vi "MW Chop PG FG.vi"() -> ()   [LabVIEW 2012]
uses:
  Microwave.lvclass
  Function Generator/Function Generator.lvclass
  Pulse Gen/Pulse Generator.lvclass
  Function Generator/Tektronix AFG 3000 Series/controls.llb/Channel.ctl
  Function Generator/Tektronix AFG 3000 Series/controls.llb/Frequency Mode.ctl
  Function Generator/Tektronix AFG 3000 Series/controls.llb/Waveform Shape.ctl
  Function Generator/Tektronix AFG 3000 Series/controls.llb/Volt Unit.ctl
  Function Generator/Tektronix AFG 3000 Series/controls.llb/Voltage.ctl
  Agilent PSG MXG Series/Agilent PSG MXG Series.lvlib
  Function Generator/Tektronix AFG 3000 Series/Tektronix AFG 3000 Series.lvlib
panel:
  in  "Enable/disable settings":bool
  in  "Copy actual to set":bool
  in  "Populate fields with member data":bool
  out "error out":errorcluster
  in  "error in (no error)":errorcluster
  in  "PG Ch 2 Sync":bool
  in  "PG Ch 1 Sync":bool
  in  "PG ch2Not rf on":bool caption="PG CH2 Not"
  in  "PG ch1Not rf on":bool caption="PG CH1 Not"
  in  "PG ch2 rf on":bool caption="PG CH2"
  in  "PG ch1 rf on":bool caption="PG CH1"
  in  "FG ch2 rf on":bool caption="FG CH2"
  in  "FG--PG":bool
  in  "FG chop freq set":dbl[unit] caption="Chop Freq."
  in  "FG volt on set":dbl[unit]=2.5 caption="On Voltage"
  in  "FG volt off set":dbl[unit] caption="Off Voltage"
  out "FG chop freq":dbl[unit] caption="Chop Freq."
  out "FG volt on":dbl[unit] caption="On Voltage"
  out "FG volt off":dbl[unit] caption="Off Voltage"
  in  "setFG":bool
  in  "FG channel":enum16{"1", "2"}(ring) caption="Channel"
  in  "FG ch1 rf on":bool caption="FG CH1"
  in  "PG chop freq set":dbl[unit]=10000.0 caption="Chop Freq."
  in  "PG volt on set":dbl[unit]=2.5 caption="On Voltage" min=-2.05 max=4.0 step=0.01
  in  "PG volt off set":dbl[unit] caption="Off Voltage" min=-2.1 max=3.95 step=0.01
  out "PG chop freq":dbl[unit] caption="Chop Freq."
  out "PG volt on":dbl[unit] caption="On Voltage"
  out "PG volt off":dbl[unit] caption="Off Voltage"
  in  "setPG":bool
  in  "PG channel":enum16{"n/a", "1", "2"}(ring)=enum."1" caption="Channel"
  in  "PG length/duty set":dbl=50.0 caption="PG pulse length/duty cycle"
  in  "PG length/duty unit set":enum16{"ns", "us", "ms", "% (duty)"}(ring)=enum."% (duty)"
  out "PG length/duty":dbl
  out "PG length/duty unit":enum16{"ns", "us", "ms", "% (duty)"}(ring)=enum."% (duty)"
  in  "readcontrol":bool
  in  "setMW":bool
  out "FG on?":bool caption="FG"
  in  "MW rf on":bool caption="MWave On/Off"
  out "MW amp":dbl=25.0 caption="MW Amp (dBm)"
  in  "MW amp set":dbl=-135.0 caption="MW Amp (dBm)"
  out "MW freq":dbl[unit] caption="MW Freq"
  in  "MW freq set":dbl[unit]=8500000000.0 caption="MW Freq"
  out "MW on?":bool caption="MW"
  out "active":bool
  in  "connect":bool
  out "PG on?":bool caption="PG"
  in  "exit":bool
  in  "read":bool
  # "Microwave Modulation"
  # "Set Chop via Pulse Generator or Function Generator and PIN Diode"
  # "Pulse Generator"
  # "Function Generator"
  # "(ready when\nblinking)"
  # "Outputs"
  # "Outputs"
  # "Microwaves"
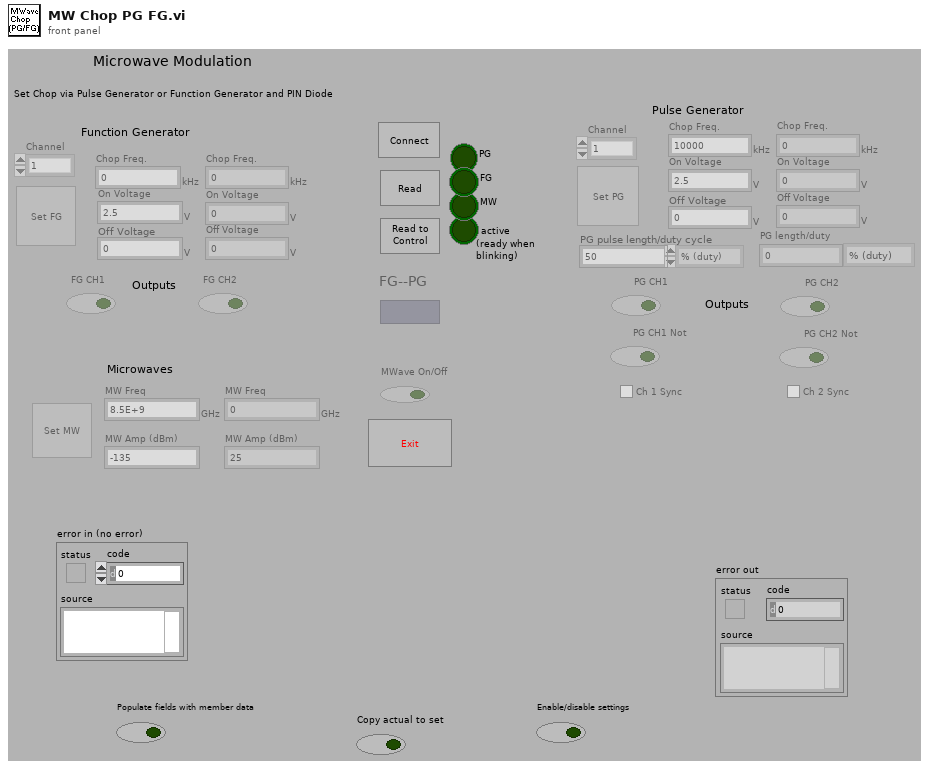
[diagram p1: front panel]
types:
  T1 = enum16{"CW", "Fixed", "Stepped Sweep", "List Sweep"}
  T2 = typedef "Voltage.ctl" = enum16{"amplitude", "offset", "high", "low", "high limit", "low limit"}
  T3 = typedef "Volt Unit.ctl" = enum16{"VPP", "VRMS", "DBM"}
  T4 = typedef "Frequency Mode.ctl" = enum16{"CW", "Sweep"}
  T5 = typedef "Channel.ctl" = u16
  T6 = typedef "Waveform Shape.ctl" = u16
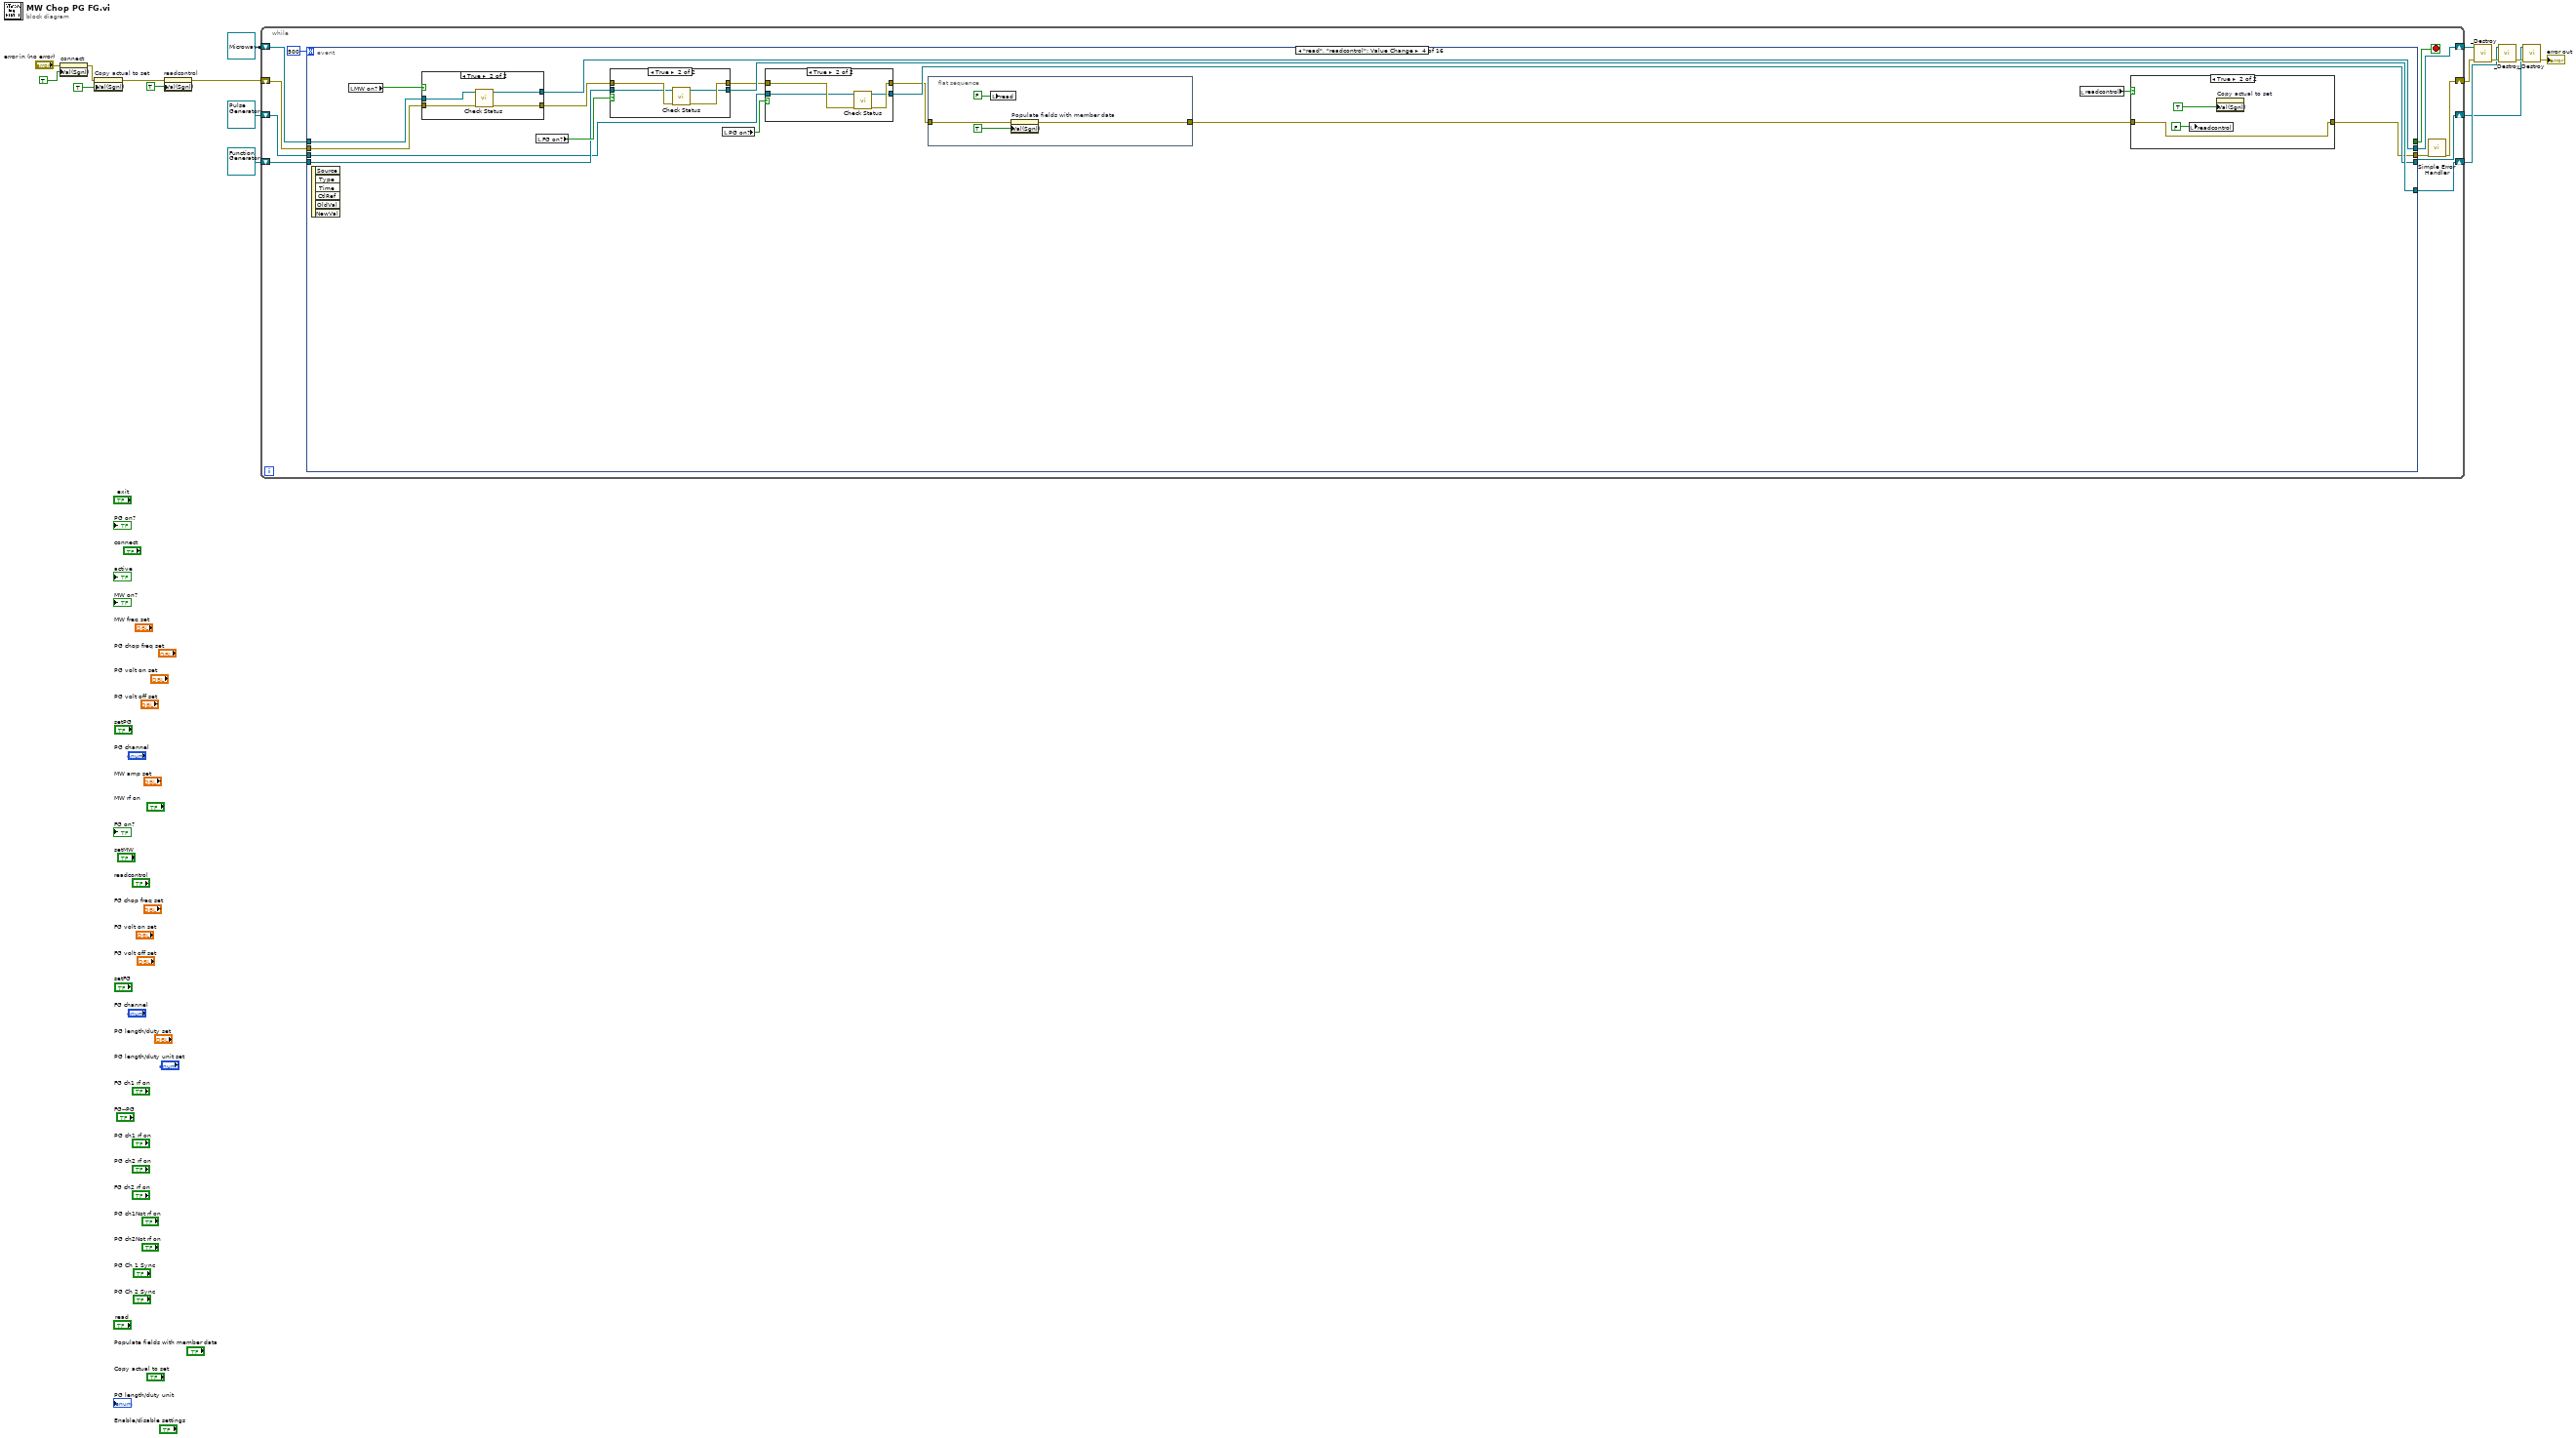
[diagram p0: block diagram]
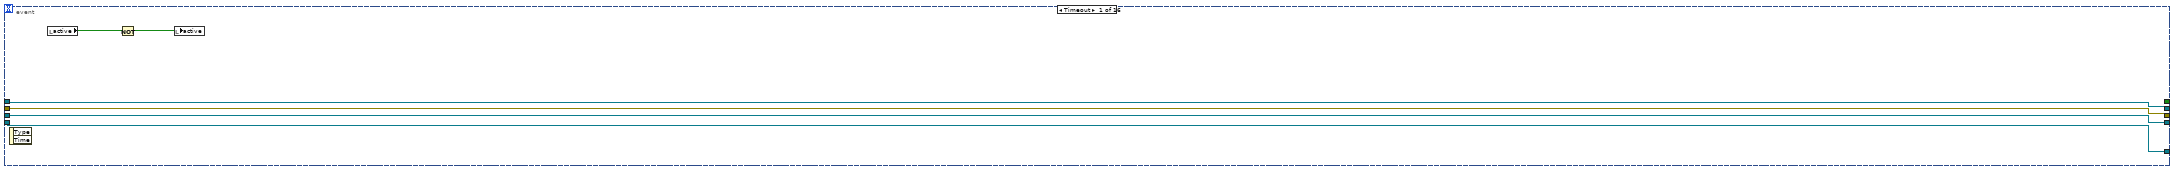
[diagram p2: hidden frame]
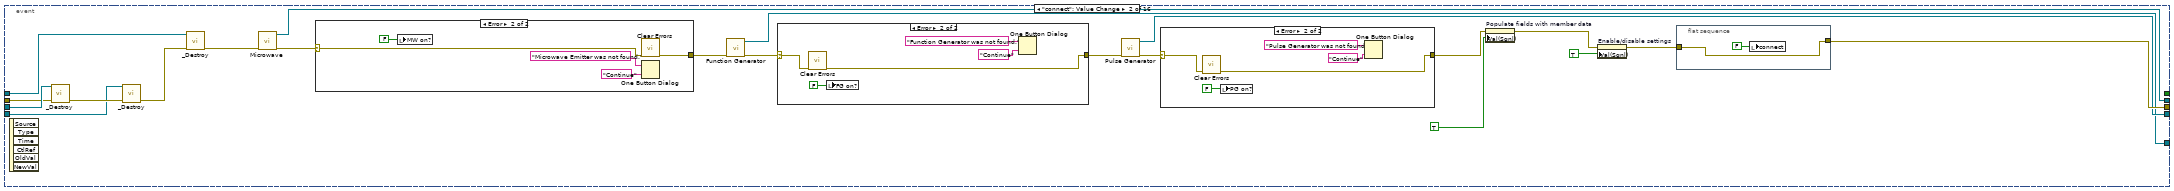
[diagram p3: hidden frame]
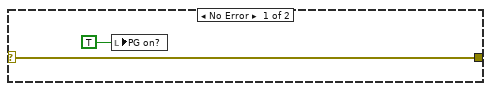
[diagram p4: hidden frame]
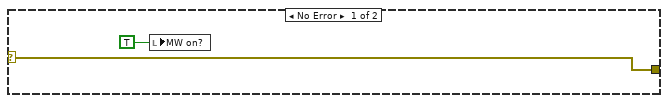
[diagram p5: hidden frame]
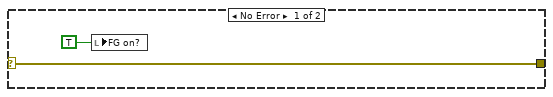
[diagram p6: hidden frame]
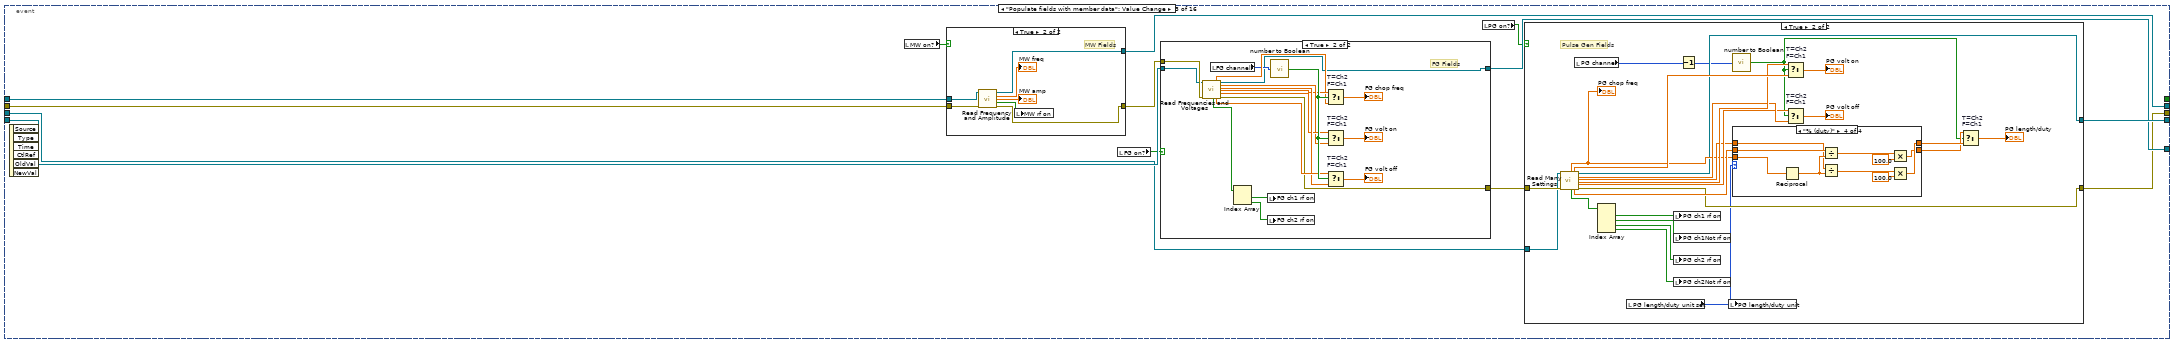
[diagram p7: hidden frame]
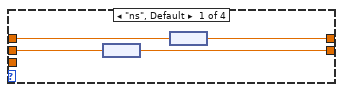
[diagram p9: hidden frame]
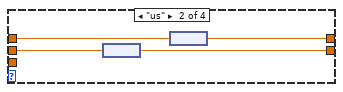
[diagram p10: hidden frame]
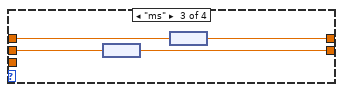
[diagram p11: hidden frame]
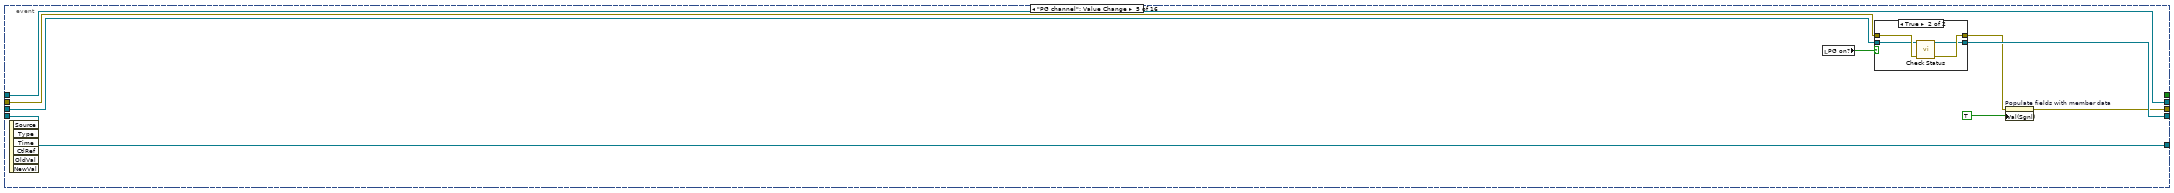
[diagram p18: hidden frame]
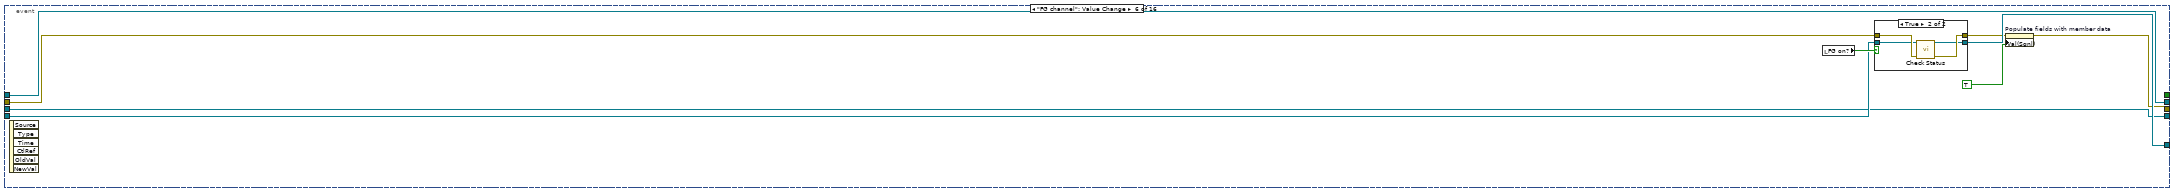
[diagram p20: hidden frame]
diagram:
  n1 = property on="connect" class="Bool (strict)"(error in="error in (no error)", "Val(Sgnl)"=TRUE ("Value (Signaling)")) -> (error out=w12:errorcluster)  [unwired: 1 in, 1 out]
  n2 = property on="Copy actual to set" class="Bool (strict)"(error in=w12, "Val(Sgnl)"=TRUE ("Value (Signaling)")) -> (error out=w3:errorcluster)  [unwired: 1 in, 1 out]
  n3 = property on="readcontrol" class="Bool (strict)"(error in=w3, "Val(Sgnl)"=TRUE ("Value (Signaling)")) -> (error out=w2:errorcluster)  [unwired: 1 in, 1 out]
  n4 = while {
    shift-right: [w21] -> w4
    shift-left: w2 -> [w22]
    shift-right: [w19] -> w7
    shift-left: refnum<class "Microwave.lvclass"> refnum ("Microwave out") -> [w25]
    shift-right: [w18] -> w6
    shift-left: refnum<class "Function Generator.lvclass"> refnum ("Function Generator out") -> [w24]
    shift-right: [w20] -> w5
    shift-left: refnum<class "Pulse Generator.lvclass"> refnum ("Pulse Generator out") -> [w23]
    stop <- w26 stop-if-true
    n5 = event shown="[3] \"read\", \"readcontrol\": Value Change" {
      selector: _ -> [_ _ _ _ _ _ _ _ _ _ _ _ _ _ _ _]
      dyn-events: _ -> [_ _ _ _ _ _ _ _ _ _ _ _ _ _ _ _]
      timeout: 500 -> [_ _ _ _ _ _ _ _ _ _ _ _ _ _ _ _]
      tunnel: w22 -> [w29 w43 w89 w181 w214 w232 w245 w267 w291 w310 w332 w360 w458 w497 w501 w520]
      tunnel: [w29 w41 w84 w170 w216 w227 w245 w258 w273 w309 w331 w365 w453 w497 w498 w520] -> w27
      tunnel: [_ _ _ _ _ _ _ _ _ _ _ _ _ TRUE ("exit") _ _] -> w26
      tunnel: w25 -> [w32 w45 w90 w182 w215 w231 w244 w262 w300 w328 w330 w362 w457 w496 w507 w519]
      tunnel: w24 -> [w31 w46 w88 w178 w213 w234 w243 w272 w297 w327 w334 w364 w455 w495 w506 w518]
      tunnel: w23 -> [w30 w47 w87 w175 w219 w229 w242 w271 w299 w312 w333 w361 w456 w494 w505 w517]
      tunnel: [w32 w39 w91 w180 w215 w231 w244 w257 w300 w328 w329 w362 w457 w496 w507 w519] -> w19
      tunnel: [w31 w38 w85 w177 w213 w233 w243 w272 w275 w327 w334 w364 w454 w495 w506 w518] -> w18
      tunnel: [w30 w40 w86 w174 w218 w229 w242 w271 w299 w311 w333 w359 w456 w494 w505 w517] -> w20
      event Timeout {
        n6 = event-data() -> ()  [unwired: 3 out]
        n7 = local read "active"() -> (w33:bool)
        n8 = Not(x=w33) -> (.not. x?=w34:bool)
        n9 = local write "active"(w34) -> ()
      }
      event "connect": Value Change {
        n10 = event-data() -> ()  [unwired: 7 out]
        n11 = call-dynamic "_Destroy.vi"("error in (no error)"=w43, "Instrument in"=w47) -> ("error out"=w50:errorcluster)  [unwired: 9 out]
        n12 = call-dynamic "_Destroy.vi"("error in (no error)"=w50, "Instrument in"=w46) -> ("error out"=w49:errorcluster)  [unwired: 9 out]
        n13 = call-dynamic "_Destroy.vi"("error in (no error)"=w49, "Instrument in"=w45) -> ("error out"=w48:errorcluster)  [unwired: 9 out]
        n14 = call "Microwave.vi"("error in (no error)"=w48) -> ("error out"=w51:errorcluster, "Microwave out"=w39:refnum<class "Microwave.lvclass">)  [unwired: 9 out]
        n15 = case shown="Error" w51 {
          selector: w51 -> [w65 w70]
          tunnel: [w65 w69] -> w54
          frame No Error {
            n16 = local write "MW on?"(TRUE ("FGon")) -> ()
          }
          frame Error {
            n17 = local write "MW on?"(FALSE ("FGon")) -> ()
            n18 = call <vilib>:"Clear Errors.vi"("error in (no error)"=w70) -> ("error out"=w69:errorcluster)  [unwired: 6 out]
            n19 = One Button Dialog(message="Microwave Emitter was not found.", button name ("OK")="Continue") -> ()  [unwired: 1 out]
          }
        }
        n20 = call "Function Generator.vi"("error in (no error)"=w54) -> ("error out"=w52:errorcluster, "Function Generator out"=w38:refnum<class "Function Generator.lvclass">)  [unwired: 9 out]
        n21 = case shown="Error" w52 {
          selector: w52 -> [w72 w77]
          tunnel: [w72 w76] -> w55
          frame No Error {
            n22 = local write "FG on?"(TRUE ("FGon")) -> ()
          }
          frame Error {
            n23 = call <vilib>:"Clear Errors.vi"("error in (no error)"=w77) -> ("error out"=w76:errorcluster)  [unwired: 6 out]
            n24 = local write "FG on?"(FALSE ("FGon")) -> ()
            n25 = One Button Dialog(message="Function Generator was not found.", button name ("OK")="Continue") -> ()  [unwired: 1 out]
          }
        }
        n26 = call "Pulse Generator.vi"("error in (no error)"=w55) -> ("error out"=w53:errorcluster, "Pulse Generator out"=w40:refnum<class "Pulse Generator.lvclass">)  [unwired: 9 out]
        n27 = case shown="Error" w53 {
          selector: w53 -> [w58 w63]
          tunnel: [w58 w62] -> w36
          frame No Error {
            n28 = local write "PG on?"(TRUE ("FGon")) -> ()
          }
          frame Error {
            n29 = call <vilib>:"Clear Errors.vi"("error in (no error)"=w63) -> ("error out"=w62:errorcluster)  [unwired: 6 out]
            n30 = local write "PG on?"(FALSE ("FGon")) -> ()
            n31 = One Button Dialog(message="Pulse Generator was not found.", button name ("OK")="Continue") -> ()  [unwired: 1 out]
          }
        }
        n32 = property on="Populate fields with member data" class="Bool (strict)"(error in=w36, "Val(Sgnl)"=TRUE ("Value (Signaling)")) -> (error out=w37:errorcluster)  [unwired: 1 in, 1 out]
        n33 = property on="Enable/disable settings" class="Bool (strict)"(error in=w37, "Val(Sgnl)"=TRUE ("Value (Signaling)")) -> (error out=w42:errorcluster)  [unwired: 1 in, 1 out]
        n34 = flat-sequence {
          tunnel: [w56] -> w41
          tunnel: w42 -> [w56]
          frame #0 {
            n35 = local write "connect"(FALSE) -> ()
          }
        }
      }
      event "Populate fields with member data": Value Change {
        n36 = event-data() -> ()  [unwired: 7 out]
        n37 = local read "MW on?"() -> (w81:bool)
        n38 = case shown="True" w81 {
          tunnel: w90 -> [w162 w163]
          tunnel: w89 -> [w161 w167]
          tunnel: [w161 w164] -> w83
          tunnel: [w162 w166] -> w91
          frame False {
          }
          frame True {
            # "MW Fields"
            n39 = call-dynamic "Read Frequency and Amplitude.vi"("Microwave.lvclass in"=w163, "error in (no error)"=w167) -> ("Microwave.lvclass out"=w166:refnum<class "Microwave.lvclass">, "Frequency"=→"MW freq":dbl[unit], "Amplitude (dBm)"=→"MW amp":dbl, "rf on?"=w165:bool, "error out"=w164:errorcluster)  [unwired: 9 out]
            n40 = local write "MW rf on"(w165) -> ()
          }
        }
        n41 = local read "FG on?"() -> (w80:bool)
        n42 = case shown="True" w80 {
          tunnel: w83 -> [w142 w149]
          tunnel: [w142 w148] -> w82
          tunnel: [w141 w147] -> w85
          tunnel: w88 -> [w141 w146]
          frame False {
          }
          frame True {
            # "FG Fields"
            n43 = call-dynamic "Read Frequencies and Voltages.vi"("Function Generator.lvclass in"=w146, "error in (no error)"=w149) -> ("array of outputs on"=w145:bool[], "Ch1 Frequency"=w151:dbl[unit], "Ch2 Low"=w158:dbl[unit], "Function Generator.lvclass out"=w147:refnum<class "Function Generator.lvclass">, "Ch1 High"=w154:dbl[unit], "Ch1 Low"=w157:dbl[unit], "Ch2 Frequency"=w152:dbl[unit], "Ch2 High"=w155:dbl[unit], "error out"=w148:errorcluster)  [unwired: 9 out]
            n44 = local read "FG channel"() -> (w150:enum16{"1", "2"})
            n45 = Index Array(array=w145) -> (element #1=w144:bool, element #2=w143:bool)  [unwired: 2 in]
            n46 = local write "FG ch1 rf on"(w144) -> ()
            n47 = local write "FG ch2 rf on"(w143) -> ()
            n48 = call "number to Boolean.vi"("Numeric"=w150) -> ("Boolean"=w159:bool)
            n49 = Select "T=Ch2\nF=Ch1"(t=w152, s=w159, f=w151) -> (s? t:f=→"FG chop freq":dbl[unit])
            n50 = Select "T=Ch2\nF=Ch1"(t=w155, s=w159, f=w154) -> (s? t:f=→"FG volt on":dbl[unit])
            n51 = Select "T=Ch2\nF=Ch1"(t=w158, s=w159, f=w157) -> (s? t:f=→"FG volt off":dbl[unit])
          }
        }
        n52 = local read "PG on?"() -> (w79:bool)
        n53 = case shown="True" w79 {
          tunnel: w82 -> [w92 w104]
          tunnel: [w92 w103] -> w84
          tunnel: w87 -> [w93 w96]
          tunnel: [w93 w102] -> w86
          frame False {
          }
          frame True {
            # "Pulse Gen Fields"
            n54 = call-dynamic "Read Many Settings.vi"("Pulse Generator.lvclass in"=w96, "error in (no error)"=w104) -> ("Overall Frequency"=w105:dbl[unit], "Outputs 1/!1/2/!2"=w97:bool[], "Output Levels.1 High"=w117:dbl[unit], "Ch2Width"=w108:dbl[unit], "Pulse Generator.lvclass out"=w102:refnum<class "Pulse Generator.lvclass">, "Output Levels.1 Low"=w114:dbl[unit], "Ch1Width"=w110:dbl[unit], "Output Levels.2 High"=w116:dbl[unit], "Output Levels.2 Low"=w113:dbl[unit], "error out"=w103:errorcluster)  [unwired: 8 out]
            "PG chop freq" <- w105
            n55 = local read "PG channel"() -> (w118:enum16{"n/a", "1", "2"})
            n56 = Index Array(array=w97) -> (element #1=w101:bool, element #2=w100:bool, element #3=w99:bool, element #4=w98:bool)  [unwired: 4 in]
            n57 = local read "PG length/duty unit set"() -> (w95:enum16{"ns", "us", "ms", "% (duty)"})
            n58 = local write "PG ch1 rf on"(w101) -> ()
            n59 = local write "PG ch1Not rf on"(w100) -> ()
            n60 = local write "PG ch2 rf on"(w99) -> ()
            n61 = local write "PG ch2Not rf on"(w98) -> ()
            n62 = Decrement(x=w118) -> (x-1=w94:enum16{"n/a", "1", "2"})
            n63 = local write "PG length/duty unit"(w95) -> ()
            n64 = call "number to Boolean.vi"("Numeric"=w94) -> ("Boolean"=w106:bool)
            n65 = case shown="\"% (duty)\"" w95 {
              tunnel: [w121 w124 w127 w132] -> w111
              tunnel: w110 -> [w122 w125 w128 w135]
              tunnel: w108 -> [w120 w126 w130 w137]
              tunnel: [w119 w123 w129 w131] -> w107
              tunnel: w105 -> [_ _ _ w140]
              frame "ns", Default {
                n66 = node(w120) -> (w119:dbl)
                n67 = node(w122) -> (w121:dbl)
              }
              frame "us" {
                n68 = node(w126) -> (w123:dbl)
                n69 = node(w125) -> (w124:dbl)
              }
              frame "ms" {
                n70 = node(w130) -> (w129:dbl)
                n71 = node(w128) -> (w127:dbl)
              }
              frame "% (duty)" {
                n72 = Reciprocal(x=w140) -> (1/x=w136:dbl[unit])
                n73 = Divide(x=w137, y=w136) -> (x/y=w138:dbl)
                n74 = Divide(x=w135, y=w136) -> (x/y=w133:dbl)
                n75 = Multiply(x=w138, y=100.0) -> (x*y=w131:dbl)
                n76 = Multiply(x=w133, y=100.0) -> (x*y=w132:dbl)
              }
            }
            n77 = Select "T=Ch2\nF=Ch1"(t=w116, s=w106, f=w117) -> (s? t:f=→"PG volt on":dbl[unit])
            n78 = Select "T=Ch2\nF=Ch1"(t=w113, s=w106, f=w114) -> (s? t:f=→"PG volt off":dbl[unit])
            n79 = Select "T=Ch2\nF=Ch1"(t=w107, s=w106, f=w111) -> (s? t:f=→"PG length/duty":dbl)
          }
        }
      }
      event "read", "readcontrol": Value Change {
        n80 = event-data() -> ()  [unwired: 7 out]
        n81 = local read "MW on?"() -> (w185:bool)
        n82 = case shown="True" w185 {
          tunnel: w182 -> [w206 w211]
          tunnel: w181 -> [w207 w210]
          tunnel: [w206 w209] -> w180
          tunnel: [w207 w208] -> w179
          frame False {
          }
          frame True {
            n83 = call-dynamic "Check Status.vi"("error in (no error)"=w210, "Microwave in"=w211) -> ("error out"=w208:errorcluster, "Microwave out"=w209:refnum<class "Microwave.lvclass">)  [unwired: 8 out]
          }
        }
        n84 = local read "FG on?"() -> (w184:bool)
        n85 = case shown="True" w184 {
          tunnel: w179 -> [w200 w205]
          tunnel: [w200 w204] -> w176
          tunnel: w178 -> [w201 w203]
          tunnel: [w201 w202] -> w177
          frame False {
          }
          frame True {
            n86 = call-dynamic "Check Status.vi"("error in (no error)"=w205, "Function Generator in"=w203) -> ("error out"=w204:errorcluster, "Function Generator out"=w202:refnum<class "Function Generator.lvclass">)  [unwired: 8 out]
          }
        }
        n87 = local read "PG on?"() -> (w183:bool)
        n88 = case shown="True" w183 {
          tunnel: w176 -> [w194 w199]
          tunnel: [w194 w198] -> w173
          tunnel: w175 -> [w195 w197]
          tunnel: [w195 w196] -> w174
          frame False {
          }
          frame True {
            n89 = call-dynamic "Check Status.vi"("error in (no error)"=w199, "Pulse Generator in"=w197) -> ("error out"=w198:errorcluster, "Pulse Generator out"=w196:refnum<class "Pulse Generator.lvclass">)  [unwired: 8 out]
          }
        }
        n90 = flat-sequence {
          tunnel: w173 -> [w193]
          tunnel: [w190] -> w171
          frame #0 {
            n91 = local write "read"(FALSE ("read")) -> ()
            n92 = property on="Populate fields with member data" class="Bool (strict)"(error in=w193, "Val(Sgnl)"=TRUE ("Value (Signaling)")) -> (error out=w190:errorcluster)  [unwired: 1 in, 1 out]
          }
        }
        n93 = local read "readcontrol"() -> (w172:bool)
        n94 = case shown="True" w172 {
          tunnel: [w186 w187] -> w170
          tunnel: w171 -> [w186 w187]
          frame False {
          }
          frame True {
            n95 = local write "readcontrol"(FALSE ("readcontrol")) -> ()
            n96 = property on="Copy actual to set" class="Bool (strict)"("Val(Sgnl)"=TRUE ("Value (Signaling)")) -> ()  [unwired: 2 in, 2 out]
          }
        }
      }
      event "PG channel": Value Change {
        n97 = event-data() -> ()  [unwired: 7 out]
        n98 = local read "PG on?"() -> (w220:bool)
        n99 = case shown="True" w220 {
          tunnel: w214 -> [w221 w226]
          tunnel: [w221 w225] -> w217
          tunnel: w219 -> [w222 w224]
          tunnel: [w222 w223] -> w218
          frame False {
          }
          frame True {
            n100 = call-dynamic "Check Status.vi"("error in (no error)"=w226, "Pulse Generator in"=w224) -> ("error out"=w225:errorcluster, "Pulse Generator out"=w223:refnum<class "Pulse Generator.lvclass">)  [unwired: 8 out]
          }
        }
        n101 = property on="Populate fields with member data" class="Bool (strict)"(error in=w217, "Val(Sgnl)"=TRUE ("Value (Signaling)")) -> (error out=w216:errorcluster)  [unwired: 1 in, 1 out]
      }
      event "FG channel": Value Change {
        n102 = event-data() -> ()  [unwired: 7 out]
        n103 = local read "FG on?"() -> (w235:bool)
        n104 = case shown="True" w235 {
          tunnel: w232 -> [w236 w241]
          tunnel: [w236 w240] -> w230
          tunnel: w234 -> [w237 w239]
          tunnel: [w237 w238] -> w233
          frame False {
          }
          frame True {
            n105 = call-dynamic "Check Status.vi"("error in (no error)"=w241, "Function Generator in"=w239) -> ("error out"=w240:errorcluster, "Function Generator out"=w238:refnum<class "Function Generator.lvclass">)  [unwired: 8 out]
          }
        }
        n106 = property on="Populate fields with member data" class="Bool (strict)"(error in=w230, "Val(Sgnl)"=TRUE ("Value (Signaling)")) -> (error out=w227:errorcluster)  [unwired: 1 in, 1 out]
      }
      event "Copy actual to set": Value Change {
        n107 = event-data() -> ()  [unwired: 7 out]
        n108 = flat-sequence {
          frame #0 {
            n109 = local read "MW freq"() -> (w246:dbl[unit])
            n110 = local read "MW amp"() -> (w247:dbl)
            n111 = local write "MW freq set"(w246) -> ()
            n112 = local write "MW amp set"(w247) -> ()
          }
          frame #1 {
            n113 = local read "FG chop freq"() -> (w250:dbl[unit])
            n114 = local read "FG volt off"() -> (w248:dbl[unit])
            n115 = local read "FG volt on"() -> (w249:dbl[unit])
            n116 = local write "FG chop freq set"(w250) -> ()
            n117 = local write "FG volt on set"(w249) -> ()
            n118 = local write "FG volt off set"(w248) -> ()
          }
          frame #2 {
            n119 = local read "PG length/duty"() -> (w254:dbl)
            n120 = local read "PG chop freq"() -> (w251:dbl[unit])
            n121 = local read "PG volt off"() -> (w252:dbl[unit])
            n122 = local read "PG volt on"() -> (w253:dbl[unit])
            n123 = local read "PG length/duty unit"() -> (w255:enum16{"ns", "us", "ms", "% (duty)"})
            n124 = local write "PG volt off set"(w252) -> ()
            n125 = local write "PG length/duty set"(w254) -> ()
            n126 = local write "PG chop freq set"(w251) -> ()
            n127 = local write "PG volt on set"(w253) -> ()
            n128 = local write "PG length/duty unit set"(w255) -> ()
          }
        }
      }
      event "MW rf on": Value Change {
        n129 = event-data() -> ("NewVal"=w261:bool)  [unwired: 6 out]
        n130 = call-dynamic "VISA Get Session.vi"("error in (no error)"=w267, "Instrument.lvclass in"=w262) -> ("error out"=w270:errorcluster, "VISA Resource Name"=w266:refnum<visa-resource-name>, "Instrument.lvclass out"=w263:refnum<class "Microwave.lvclass">)  [unwired: 7 out]
        n131 = call "Set Output.vi"("error in (no error)"=w270, "Output On"=w261, "VISA resource name"=w266) -> ("error out"=w269:errorcluster, "VISA resource name out"=w265:refnum<visa-resource-name>)  [unwired: 7 out]
        n132 = call "Query Output.vi"("error in (no error)"=w269, "VISA resource name"=w265) -> ("error out"=w268:errorcluster, "Output On?"=w260:bool, "VISA resource name out"=w264:refnum<visa-resource-name>)  [unwired: 7 out]
        n133 = local write "MW rf on"(w260) -> ()
        n134 = call-dynamic "VISA Save Session.vi"("error in (no error)"=w268, "VISA Resource Name"=w264, "Instrument.lvclass in"=w263) -> ("error out"=w259:errorcluster, "Instrument.lvclass out"=w256:refnum<class "Microwave.lvclass">)  [unwired: 7 out]
        n135 = call-dynamic "Set member data - output.vi"("error in (no error)"=w259, "rf on?"=w260, "Microwave.lvclass in"=w256) -> ("error out"=w258:errorcluster, "Microwave.lvclass out"=w257:refnum<class "Microwave.lvclass">)  [unwired: 7 out]
      }
      event "FG ch1 rf on", "FG ch2 rf on": Value Change {
        w282 = T5 1 items=["Channel 1", "Channel 2"] ("Channel (0: Channel 1)")
        w283 = T5 1 items=["Channel 1", "Channel 2"] ("Channel (0: Channel 1)")
        w284 = T5 0 items=["Channel 1", "Channel 2"] ("Channel (0: Channel 1)")
        w285 = T5 0 items=["Channel 1", "Channel 2"] ("Channel (0: Channel 1)")
        n136 = event-data() -> ()  [unwired: 7 out]
        n137 = local read "FG ch1 rf on"() -> (w281:bool)
        n138 = call-dynamic "VISA Get Session.vi"("error in (no error)"=w291, "Instrument.lvclass in"=w297) -> ("error out"=w296:errorcluster, "VISA Resource Name"=w290:refnum<visa-resource-name>, "Instrument.lvclass out"=w298:refnum<class "Function Generator.lvclass">)  [unwired: 7 out]
        n139 = call "Enable Output.vi"("Enable Output (T: Enable)"=w281, "error in (no error)"=w296, "Channel (0: Channel 1)"=w285, "VISA resource name"=w290) -> ("error out"=w295:errorcluster, "VISA resource name out"=w289:refnum<visa-resource-name>)  [unwired: 6 out]
        n140 = local read "FG ch2 rf on"() -> (w280:bool)
        n141 = call "Query Output.vi"("error in (no error)"=w295, "Channel (0: Channel 1)"=w284, "VISA resource name"=w289) -> ("error out"=w294:errorcluster, "Output Enabled?"=w279:bool, "VISA resource name out"=w288:refnum<visa-resource-name>)  [unwired: 6 out]
        n142 = local write "FG ch1 rf on"(w279) -> ()
        n143 = call "Enable Output.vi"("Enable Output (T: Enable)"=w280, "error in (no error)"=w294, "Channel (0: Channel 1)"=w283, "VISA resource name"=w288) -> ("error out"=w293:errorcluster, "VISA resource name out"=w287:refnum<visa-resource-name>)  [unwired: 6 out]
        n144 = call "Query Output.vi"("error in (no error)"=w293, "Channel (0: Channel 1)"=w282, "VISA resource name"=w287) -> ("error out"=w292:errorcluster, "Output Enabled?"=w278:bool, "VISA resource name out"=w286:refnum<visa-resource-name>)  [unwired: 6 out]
        n145 = local write "FG ch2 rf on"(w278) -> ()
        n146 = call-dynamic "VISA Save Session.vi"("error in (no error)"=w292, "VISA Resource Name"=w286, "Instrument.lvclass in"=w298) -> ("error out"=w274:errorcluster, "Instrument.lvclass out"=w276:refnum<class "Function Generator.lvclass">)  [unwired: 7 out]
        n147 = Build Array(w279, w278) -> (w277:bool[])
        n148 = call-dynamic "Set member data - outputs on.vi"("error in (no error)"=w274, "Array of outputs on?"=w277, "Function Generator.lvclass in"=w276) -> ("error out"=w273:errorcluster, "Function Generator.lvclass out"=w275:refnum<class "Function Generator.lvclass">)  [unwired: 7 out]
      }
      event "PG ch1 rf on", "PG ch1Not rf on", "PG ch2 rf on", "PG ch2Not rf on": Value Change {
        n149 = event-data() -> ()  [unwired: 7 out]
        n150 = local read "PG ch1Not rf on"() -> (w306:bool)
        n151 = local read "PG ch2Not rf on"() -> (w302:bool)
        n152 = local read "PG Ch 1 Sync"() -> (w308:bool)
        n153 = local read "PG Ch 2 Sync"() -> (w304:bool)
        n154 = local read "PG ch1 rf on"() -> (w305:bool)
        n155 = local read "PG ch2 rf on"() -> (w301:bool)
        n156 = Select(t=w305, s=w308, f=w306) -> (s? t:f=w307:bool)
        n157 = Select(t=w301, s=w304, f=w302) -> (s? t:f=w303:bool)
        n158 = call-dynamic "VISA Get Session.vi"("error in (no error)"=w310, "Instrument.lvclass in"=w312) -> ("error out"=w322:errorcluster, "VISA Resource Name"=w325:refnum<visa-resource-name>, "Instrument.lvclass out"=w326:refnum<class "Pulse Generator.lvclass">)  [unwired: 7 out]
        n159 = call "HP81110A Output Set - Fast.vi"("notoutput2"=w303, "output1"=w305, "error in (no error)"=w322, "output2"=w301, "notoutput1"=w307, "VISA session"=w325) -> ("error out"=w321:errorcluster, "dup VISA session"=w324:refnum<visa-resource-name>)  [unwired: 4 out]
        n160 = call "HP81110A Output Get.vi"("error in (no error)"=w321, "VISA session"=w324) -> ("error out"=w320:errorcluster, "output2OUT"=w317:bool, "notoutput1OUT"=w318:bool, "dup VISA session"=w323:refnum<visa-resource-name>, "notoutput2OUT"=w316:bool, "output1OUT"=w319:bool)  [unwired: 4 out]
        n161 = local write "PG ch1 rf on"(w319) -> ()
        n162 = local write "PG ch1Not rf on"(w318) -> ()
        n163 = local write "PG ch2 rf on"(w317) -> ()
        n164 = local write "PG ch2Not rf on"(w316) -> ()
        n165 = Build Array(w319, w318, w317, w316) -> (w315:bool[])
        n166 = call-dynamic "VISA Save Session.vi"("error in (no error)"=w320, "VISA Resource Name"=w323, "Instrument.lvclass in"=w326) -> ("error out"=w313:errorcluster, "Instrument.lvclass out"=w314:refnum<class "Pulse Generator.lvclass">)  [unwired: 7 out]
        n167 = call-dynamic "Set member data - outputs on.vi"("error in (no error)"=w313, "Outputs 1/!1/2/!2"=w315, "Pulse Generator.lvclass in"=w314) -> ("error out"=w309:errorcluster, "Pulse Generator.lvclass out"=w311:refnum<class "Pulse Generator.lvclass">)  [unwired: 7 out]
      }
      event "setMW": Value Change {
        n168 = event-data() -> ()  [unwired: 7 out]
        n169 = flat-sequence {
          tunnel: w332 -> [w344]
          tunnel: w330 -> [w343]
          tunnel: [w338] -> w331
          tunnel: [w336] -> w329
          frame #0 {
            n170 = call-dynamic "VISA Get Session.vi"("error in (no error)"=w344, "Instrument.lvclass in"=w343) -> ("error out"=w357:errorcluster, "VISA Resource Name"=w355:refnum<visa-resource-name>, "Instrument.lvclass out"=w356:refnum<class "Microwave.lvclass">)  [unwired: 7 out]
            n171 = call "Set Frequency Mode.vi"("error in (no error)"=w357, "Frequency Mode"=T1."CW", "VISA resource name"=w355) -> ("error out"=w348:errorcluster, "VISA resource name out"=w347:refnum<visa-resource-name>)  [unwired: 7 out]
            n172 = local read "MW freq set"() -> (w350:dbl[unit])
            n173 = call "Set Amplitude Mode.vi"("error in (no error)"=w348, "Amplitude Mode"=enum16{"Fixed", "Stepped Sweep", "List Sweep"}."Fixed", "VISA resource name"=w347) -> ("error out"=w351:errorcluster, "VISA resource name out"=w349:refnum<visa-resource-name>)  [unwired: 7 out]
            n174 = local read "MW amp set"() -> (w352:dbl)
            n175 = call "Set Frequency.vi"("error in (no error)"=w351, "Frequency"=w350, "VISA resource name"=w349) -> ("error out"=w353:errorcluster, "VISA resource name out"=w354:refnum<visa-resource-name>)  [unwired: 7 out]
            n176 = call "Set Amplitude.vi"("error in (no error)"=w353, "Amplitude (dBm)"=w352, "VISA resource name"=w354) -> ("error out"=w342:errorcluster, "VISA resource name out"=w341:refnum<visa-resource-name>)  [unwired: 7 out]
            n177 = call-dynamic "VISA Save Session.vi"("error in (no error)"=w342, "VISA Resource Name"=w341, "Instrument.lvclass in"=w356) -> ("error out"=w340:errorcluster, "Instrument.lvclass out"=w337:refnum<class "Microwave.lvclass">)  [unwired: 7 out]
            n178 = call-dynamic "Check Status.vi"("error in (no error)"=w340, "Microwave in"=w337) -> ("error out"=w339:errorcluster, "Microwave out"=w336:refnum<class "Microwave.lvclass">)  [unwired: 8 out]
            n179 = property on="Populate fields with member data" class="Bool (strict)"(error in=w339, "Val(Sgnl)"=TRUE ("Value (Signaling)")) -> (error out=w338:errorcluster)  [unwired: 1 in, 1 out]
          }
          frame #1 {
            n180 = local write "setMW"(FALSE) -> ()
          }
        }
      }
      event "setPG": Value Change {
        n181 = event-data() -> ()  [unwired: 7 out]
        n182 = flat-sequence {
          tunnel: [w368] -> w363
          tunnel: w361 -> [w385]
          tunnel: w360 -> [w384]
          tunnel: [w366] -> w359
          tunnel: [w451] -> w365
          tunnel: w363 -> [w451]
          frame #0 {
            n183 = local read "PG volt off set"() -> (w393:dbl[unit])
            n184 = local read "PG volt on set"() -> (w394:dbl[unit])
            n185 = call-dynamic "VISA Get Session.vi"("error in (no error)"=w384, "Instrument.lvclass in"=w385) -> ("error out"=w379:errorcluster, "VISA Resource Name"=w383:refnum<visa-resource-name>, "Instrument.lvclass out"=w382:refnum<class "Pulse Generator.lvclass">)  [unwired: 7 out]
            n186 = local read "PG chop freq set"() -> (w401:dbl[unit])
            n187 = Subtract(x=w394, y=w393) -> (x-y=w399:dbl[unit])
            n188 = call "HP81110A Generating Cont Pulses.vi"("error in (no error)"=w379, "VISA session"=w383) -> ("error out"=w403:errorcluster, "dup VISA session"=w404:refnum<visa-resource-name>)  [unwired: 2 in, 6 out]
            n189 = call "HP81110A Set Value Of Frequency.vi"("error in (no error)"=w403, "Frequency Value"=w401, "VISA session"=w404) -> ("error out"=w377:errorcluster, "dup VISA session"=w402:refnum<visa-resource-name>)  [unwired: 7 out]
            n190 = node(w399) -> (w398:dbl)
            n191 = Equal To 0?(x=w398) -> (x = 0?=w397:bool)
            n192 = case shown="True" w397 {
              tunnel: [w413 w416] -> w396
              tunnel: [w412 w417] -> w395
              tunnel: w394 -> [w413 _]
              tunnel: w393 -> [w412 _]
              tunnel: w377 -> [w411 w415]
              tunnel: [w411 w414] -> w376
              frame False {
              }
              frame True {
                # "If \"on\" and \"off\" are equal, ask for new values\nand \"Set\" again"
                n193 = call "Pulse Generator Voltage Level Error"("error in (no error)"=w415) -> ("Off Voltage"=w418:dbl, "On Voltage"=w419:dbl, "error out"=w414:errorcluster)  [unwired: 2 in, 14 out]
                n194 = node(w419) -> (w416:dbl[unit])
                n195 = node(w418) -> (w417:dbl[unit])
                n196 = local write "PG volt on set"(w416) -> ()
                n197 = local write "PG volt off set"(w417) -> ()
              }
            }
            n198 = local read "PG channel"() -> (w392:enum16{"n/a", "1", "2"})
            n199 = local read "PG chop freq set"() -> (w391:dbl[unit])
            n200 = local read "PG length/duty unit set"() -> (w367:enum16{"ns", "us", "ms", "% (duty)"})
            n201 = local read "PG length/duty set"() -> (w400:dbl)
            n202 = To Byte Integer(number=w392) -> (8bit integer=w378:i8)
            n203 = call "HP81110A Set High Low Level Of Outputs.vi"("Value Low (-0.5 V)"=w395, "error in (no error)"=w376, "Value High (0.5 V)"=w396, "Channel (1:Channel 1)"=w378, "VISA session"=w402) -> ("error out"=w374:errorcluster, "dup VISA session"=w389:refnum<visa-resource-name>)  [unwired: 5 out]
            n204 = Reciprocal(x=w391) -> (1/x=w390:dbl[unit])
            n205 = local write "PG length/duty unit"(w367) -> ()
            n206 = case shown="\"% (duty)\"" w367 {
              tunnel: w400 -> [w424 w428 w433 w437]
              tunnel: w390 -> [w423 w429 w434 w443]
              tunnel: [w422 w427 w432 FALSE] -> w388
              tunnel: [w421 w426 w431 w441] -> w387
              tunnel: w374 -> [w420 w425 w430 w439]
              tunnel: [w420 w425 w430 w438] -> w375
              frame "ns", Default {
                n207 = node(w424) -> (w421:dbl[unit])
                n208 = Less?(x=w423, y=w421) -> (x < y?=w422:bool)
              }
              frame "us" {
                n209 = node(w428) -> (w426:dbl[unit])
                n210 = Less?(x=w429, y=w426) -> (x < y?=w427:bool)
              }
              frame "ms" {
                n211 = node(w433) -> (w431:dbl[unit])
                n212 = Less?(x=w434, y=w431) -> (x < y?=w432:bool)
              }
              frame "% (duty)" {
                n213 = Divide(x=w437, y=i8 100) -> (x/y=w436:dbl)
                n214 = Greater?(x=w436, y=1) -> (0:w444:bool)
                n215 = case shown="True" w444 {
                  tunnel: [w447 w450] -> w442
                  tunnel: w436 -> [w447 _]
                  tunnel: w439 -> [w446 w449]
                  tunnel: [w446 w448] -> w438
                  frame False {
                  }
                  frame True {
                    n216 = call "Pulse Generator Duty Cycle Error"("error in (no error)"=w449) -> ("Duty Cycle"=w450:dbl, "error out"=w448:errorcluster)  [unwired: 2 in, 15 out]
                    n217 = local write "PG length/duty set"(w450) -> ()
                  }
                }
                n218 = Multiply(x=w443, y=w442) -> (x*y=w441:dbl[unit])
              }
            }
            n219 = case shown="True" w388 {
              tunnel: [w406 w410] -> w386
              tunnel: w387 -> [w406 _]
              tunnel: w375 -> [w405 w408]
              tunnel: [w405 w407] -> w373
              frame False {
              }
              frame True {
                n220 = call "Pulse Generator Pulse Length Error"("error in (no error)"=w408) -> ("Pulse Length"=w409:dbl, "error out"=w407:errorcluster)  [unwired: 2 in, 15 out]
                n221 = local write "PG length/duty set"(w409) -> ()
                n222 = node(w409) -> (w410:dbl[unit])
              }
            }
            n223 = call "HP81110A Set Value Of Width.vi"("Width Value (100.0E-9)"=w386, "error in (no error)"=w373, "Channel (1:Channel 1)"=w378, "VISA session"=w389) -> ("error out"=w380:errorcluster, "dup VISA session"=w381:refnum<visa-resource-name>)  [unwired: 1 in, 5 out]
            n224 = call-dynamic "VISA Save Session.vi"("error in (no error)"=w380, "VISA Resource Name"=w381, "Instrument.lvclass in"=w382) -> ("error out"=w369:errorcluster, "Instrument.lvclass out"=w372:refnum<class "Pulse Generator.lvclass">)  [unwired: 7 out]
            n225 = call-dynamic "Check Status.vi"("error in (no error)"=w369, "Pulse Generator in"=w372) -> ("error out"=w371:errorcluster, "Pulse Generator out"=w366:refnum<class "Pulse Generator.lvclass">)  [unwired: 8 out]
            n226 = property on="Populate fields with member data" class="Bool (strict)"(error in=w371, "Val(Sgnl)"=TRUE ("Value (Signaling)")) -> (error out=w368:errorcluster)  [unwired: 1 in, 1 out]
          }
          frame #1 {
            n227 = local write "setPG"(FALSE) -> ()
          }
        }
      }
      event "setFG": Value Change {
        n228 = event-data() -> ()  [unwired: 7 out]
        n229 = flat-sequence {
          tunnel: w458 -> [w468]
          tunnel: w455 -> [w469]
          tunnel: [w464] -> w454
          tunnel: [w461] -> w453
          frame #0 {
            w475 = T6 1 items=["Sinusoid", "Square", "Pulse", "Ramp", "PRNoise", "DC", "SINC", "Gaussian", "Lorentz", "ERise", "EDecay", "Haversine", "User 1", "User 2", "User 3", "User 4", "EMemory", "EFile"] ("Waveform Shape")
            n230 = local read "FG channel"() -> (w459:enum16{"1", "2"})
            n231 = call-dynamic "VISA Get Session.vi"("error in (no error)"=w468, "Instrument.lvclass in"=w469) -> ("error out"=w474:errorcluster, "VISA Resource Name"=w473:refnum<visa-resource-name>, "Instrument.lvclass out"=w470:refnum<class "Function Generator.lvclass">)  [unwired: 7 out]
            n232 = call "Set Frequency Mode.vi"("error in (no error)"=w474, "Mode (0: CW)"=Frequency_Mode."CW", "Channel (0: Channel 1)"=w459, "VISA resource name"=w473) -> ("error out"=w476:errorcluster, "VISA resource name out"=w466:refnum<visa-resource-name>)  [unwired: 6 out]
            n233 = local read "FG chop freq set"() -> (w490:dbl[unit])
            n234 = call "Set Waveform Shape.vi"("error in (no error)"=w476, "Waveform Shape"=w475, "Channel (0: Channel 1)"=w459, "VISA resource name"=w466) -> ("error out"=w488:errorcluster, "VISA resource name out"=w486:refnum<visa-resource-name>)  [unwired: 6 out]
            n235 = call "Set Frequency.vi"("error in (no error)"=w488, "frequency"=w490, "Channel (0: Channel 1)"=w459, "VISA resource name"=w486) -> ("error out"=w489:errorcluster, "VISA resource name out"=w487:refnum<visa-resource-name>)  [unwired: 6 out]
            n236 = local read "FG volt on set"() -> (w480:dbl[unit])
            n237 = call "Set Voltage Unit.vi"("error in (no error)"=w489, "Volt Unit (VPP)"=Volt_Unit."VPP", "Channel (0: Channel 1)"=w459, "VISA resource name"=w487) -> ("error out"=w481:errorcluster, "VISA resource name out"=w485:refnum<visa-resource-name>)  [unwired: 6 out]
            n238 = local read "FG volt off set"() -> (w483:dbl[unit])
            n239 = call "Set Voltage.vi"("Voltage Param (amplitude)"=Voltage."high", "error in (no error)"=w481, "voltage"=w480, "Channel (0: Channel 1)"=w459, "VISA resource name"=w485) -> ("error out"=w482:errorcluster, "VISA resource name out"=w484:refnum<visa-resource-name>)  [unwired: 5 out]
            n240 = call "Set Voltage.vi"("Voltage Param (amplitude)"=Voltage."low", "error in (no error)"=w482, "voltage"=w483, "Channel (0: Channel 1)"=w459, "VISA resource name"=w484) -> ("error out"=w467:errorcluster, "VISA resource name out"=w471:refnum<visa-resource-name>)  [unwired: 5 out]
            n241 = call-dynamic "VISA Save Session.vi"("error in (no error)"=w467, "VISA Resource Name"=w471, "Instrument.lvclass in"=w470) -> ("error out"=w462:errorcluster, "Instrument.lvclass out"=w465:refnum<class "Function Generator.lvclass">)  [unwired: 7 out]
            n242 = call-dynamic "Check Status.vi"("error in (no error)"=w462, "Function Generator in"=w465) -> ("error out"=w463:errorcluster, "Function Generator out"=w464:refnum<class "Function Generator.lvclass">)  [unwired: 8 out]
            n243 = property on="Populate fields with member data" class="Bool (strict)"(error in=w463, "Val(Sgnl)"=TRUE ("Value (Signaling)")) -> (error out=w461:errorcluster)  [unwired: 1 in, 1 out]
          }
          frame #1 {
            n244 = local write "setFG"(FALSE ("setFG")) -> ()
          }
        }
      }
      event "exit": Value Change {
        n245 = event-data() -> ()  [unwired: 7 out]
        n246 = local write "exit"(FALSE ("exit")) -> ()
      }
      event "FG--PG": Value Change {
        n247 = event-data() -> ()  [unwired: 7 out]
        n248 = local read "FG--PG"() -> (w504:bool)
        n249 = case shown="True" w504 {
          tunnel: w501 -> [w510 w514]
          tunnel: [w508 w512] -> w500
          frame False {
            w511 = FALSE
            # "Turns PG outputs off if switching away from PG"
            n250 = property on="PG ch1 rf on" class="Bool (strict)"(error in=w510, "Val(Sgnl)"=w511) -> (error out=w509:errorcluster)  [unwired: 1 in, 1 out]
            n251 = property on="PG ch2 rf on" class="Bool (strict)"(error in=w509, "Val(Sgnl)"=w511) -> (error out=w508:errorcluster)  [unwired: 1 in, 1 out]
          }
          frame True {
            w515 = FALSE
            # "Turns FG outputs off if switching away from FG"
            n252 = property on="FG ch1 rf on" class="Bool (strict)"(error in=w514, "Val(Sgnl)"=w515) -> (error out=w513:errorcluster)  [unwired: 1 in, 1 out]
            n253 = property on="FG ch2 rf on" class="Bool (strict)"(error in=w513, "Val(Sgnl)"=w515) -> (error out=w512:errorcluster)  [unwired: 1 in, 1 out]
          }
        }
        n254 = property on="read" class="Bool (strict)"(error in=w500, "Val(Sgnl)"=TRUE) -> (error out=w499:errorcluster)  [unwired: 1 in, 1 out]
        n255 = property on="Enable/disable settings" class="Bool (strict)"(error in=w499, "Val(Sgnl)"=TRUE ("Value (Signaling)")) -> (error out=w498:errorcluster)  [unwired: 1 in, 1 out]
      }
      event "Enable/disable settings": Value Change {
        # "Disables controls for devices not selected/turned on."
        n256 = event-data() -> ()  [unwired: 7 out]
        n257 = flat-sequence {
          tunnel: [w544] -> w516
          tunnel: w516 -> [w547]
          frame #0 {
            # "PG and FG:\nOnly enable FG-PG switch if both are one.\nIf only one is one, move the switch to the appropriate position."
            n258 = local read "PG on?"() -> (w526:bool)
            n259 = local read "FG on?"() -> (w524:bool)
            n260 = And "Both are on"(x=w524, y=w526) -> (x .and. y?=w525:bool)
            n261 = Exclusive Or "Only one on"(1:w526, 2:w524) -> (0:w527:bool)
            n262 = local read "FG--PG"() -> (w529:bool)
            n263 = Select(t=0, s=w525, f=2) -> (s? t:f=w523:i32)
            n264 = property on="FG--PG" class="Bool (strict)"("Disabled"=w523) -> ()  [unwired: 2 in, 2 out]
            n265 = Select(t=w526, s=w527, f=w529) -> (s? t:f=w528:bool)
            n266 = local write "FG--PG"(w528) -> ()
          }
          frame #1 {
            # "MW: must be on in order to enable all of these settings."
            n267 = local read "MW on?"() -> (w533:bool)
            n268 = Select(t=0, s=w533, f=2) -> (s? t:f=w530:i32)
            n269 = property on="MW rf on" class="Bool (strict)"("Disabled"=w530) -> ()  [unwired: 2 in, 2 out]
            n270 = property on="MW freq" class="DigNum (strict)"("Disabled"=w530) -> ()  [unwired: 2 in, 2 out]
            n271 = property on="setMW" class="Bool (strict)"("Disabled"=w530) -> ()  [unwired: 2 in, 2 out]
            n272 = property on="MW amp set" class="DigNum (strict)"("Disabled"=w530) -> ()  [unwired: 2 in, 2 out]
            n273 = property on="MW amp" class="DigNum (strict)"("Disabled"=w530) -> ()  [unwired: 2 in, 2 out]
            n274 = property on="MW freq set" class="DigNum (strict)"("Disabled"=w530) -> ()  [unwired: 2 in, 2 out]
          }
          frame #2 {
            # "FG: must be both on and selected by FG/PG \ntoggle in order to enable all of these settings."
            n275 = local read "FG--PG"() -> (w535:bool)
            n276 = local read "FG on?"() -> (w537:bool)
            n277 = Not(x=w535) -> (.not. x?=w534:bool)
            n278 = And(x=w534, y=w537) -> (x .and. y?=w536:bool)
            n279 = Select(t=0, s=w536, f=2) -> (s? t:f=w538:i32)
            n280 = property on="FG channel" class="Enum (strict)"("Disabled"=w538) -> ()  [unwired: 2 in, 2 out]
            n281 = property on="FG volt off" class="DigNum (strict)"("Disabled"=w538) -> ()  [unwired: 2 in, 2 out]
            n282 = property on="FG chop freq set" class="DigNum (strict)"("Disabled"=w538) -> ()  [unwired: 2 in, 2 out]
            n283 = property on="FG volt on set" class="DigNum (strict)"("Disabled"=w538) -> ()  [unwired: 2 in, 2 out]
            n284 = property on="FG chop freq" class="DigNum (strict)"("Disabled"=w538) -> ()  [unwired: 2 in, 2 out]
            n285 = property on="FG volt on" class="DigNum (strict)"("Disabled"=w538) -> ()  [unwired: 2 in, 2 out]
            n286 = property on="setFG" class="Bool (strict)"("Disabled"=w538) -> ()  [unwired: 2 in, 2 out]
            n287 = property on="FG ch1 rf on" class="Bool (strict)"("Disabled"=w538) -> ()  [unwired: 2 in, 2 out]
            n288 = property on="FG ch2 rf on" class="Bool (strict)"("Disabled"=w538) -> ()  [unwired: 2 in, 2 out]
            n289 = property on="FG volt off set" class="DigNum (strict)"("Disabled"=w538) -> ()  [unwired: 2 in, 2 out]
          }
          frame #3 {
            # "PG: must be both on and selected by FG/PG \ntoggle in order to enable all of these settings."
            n290 = local read "FG--PG"() -> (w542:bool)
            n291 = local read "PG on?"() -> (w543:bool)
            n292 = And(x=w542, y=w543) -> (x .and. y?=w541:bool)
            n293 = Select(t=0, s=w541, f=2) -> (s? t:f=w544:i32)
            n294 = property on="PG volt on set" class="DigNum (strict)"("Disabled"=w544) -> ()  [unwired: 2 in, 2 out]
            n295 = property on="PG length/duty set" class="DigNum (strict)"("Disabled"=w544) -> ()  [unwired: 2 in, 2 out]
            n296 = property on="PG volt on" class="DigNum (strict)"("Disabled"=w544) -> ()  [unwired: 2 in, 2 out]
            n297 = property on="PG ch2Not rf on" class="Bool (strict)"("Disabled"=w544) -> ()  [unwired: 2 in, 2 out]
            n298 = property on="PG ch1 rf on" class="Bool (strict)"("Disabled"=w544) -> ()  [unwired: 2 in, 2 out]
            n299 = property on="PG length/duty unit set" class="Enum (strict)"("Disabled"=w544) -> ()  [unwired: 2 in, 2 out]
            n300 = property on="PG length/duty unit" class="Enum (strict)"("Disabled"=w544) -> ()  [unwired: 2 in, 2 out]
            n301 = property on="PG Ch 1 Sync" class="Bool (strict)"("Disabled"=w544) -> ()  [unwired: 2 in, 2 out]
          }
          frame #4 {
            # "same as last frame (moved here so block \ndiagram isn't too big vertically)"
            n302 = property on="PG ch2 rf on" class="Bool (strict)"("Disabled"=w547) -> ()  [unwired: 2 in, 2 out]
            n303 = property on="PG length/duty" class="DigNum (strict)"("Disabled"=w547) -> ()  [unwired: 2 in, 2 out]
            n304 = property on="PG Ch 2 Sync" class="Bool (strict)"("Disabled"=w547) -> ()  [unwired: 2 in, 2 out]
            n305 = property on="setPG" class="Bool (strict)"("Disabled"=w547) -> ()  [unwired: 2 in, 2 out]
            n306 = property on="PG channel" class="Enum (strict)"("Disabled"=w547) -> ()  [unwired: 2 in, 2 out]
            n307 = property on="PG volt off set" class="DigNum (strict)"("Disabled"=w547) -> ()  [unwired: 2 in, 2 out]
            n308 = property on="PG chop freq set" class="DigNum (strict)"("Disabled"=w547) -> ()  [unwired: 2 in, 2 out]
            n309 = property on="PG ch1Not rf on" class="Bool (strict)"("Disabled"=w547) -> ()  [unwired: 2 in, 2 out]
            n310 = property on="PG volt off" class="DigNum (strict)"("Disabled"=w547) -> ()  [unwired: 2 in, 2 out]
            n311 = property on="PG chop freq" class="DigNum (strict)"("Disabled"=w547) -> ()  [unwired: 2 in, 2 out]
          }
        }
      }
    }
    n312 = call <vilib>:"Simple Error Handler.vi"("error in (no error)"=w27) -> ("error out"=w21:errorcluster)  [unwired: 1 in, 7 out]
  }
  n313 = call-dynamic "_Destroy.vi"("error in (no error)"=w4, "Instrument in"=w7) -> ("error out"=w16:errorcluster)  [unwired: 9 out]
  n314 = call-dynamic "_Destroy.vi"("error in (no error)"=w16, "Instrument in"=w6) -> ("error out"=w15:errorcluster)  [unwired: 9 out]
  n315 = call-dynamic "_Destroy.vi"("error in (no error)"=w15, "Instrument in"=w5) -> ("error out"=→"error out":errorcluster)  [unwired: 9 out]
